vi "Loop_SM.vi"() -> ()   [LabVIEW 2017, in "Claw_Rotation.lvlib"]
uses:
  Claw_Rotation.lvlib
  CLUSTER_CMD_SM_Lift_Rotate.ctl
  ENUM_SM_Rotate_Positions.ctl
  _SHARE ALL/TypeDef Share All/CLUSTER_TalonInput.ctl
  System Drivers/Phoenix-LabVIEW/Motor Controller/Controls/CTRE_Phoenix_MotorControl_ControlMode.ctl
  TypeDef/CLUSTER_PID.ctl
  ENUM_SM_State.ctl
  CLUSTER_ACT_Lift Output.ctl
  _SHARE ALL/RoboRio Share All/SRX Share All/TypeDefs SRX/Cluster_SRX_General Data.ctl
  _SHARE ALL/RoboRio Share All/SRX Share All/TypeDefs SRX/Cluster_SRX_Common Runtime Data.ctl
  _SHARE ALL/RoboRio Share All/SRX Share All/TypeDefs SRX/Cluster_SRX_Error Calculations.ctl
  _SHARE ALL/RoboRio Share All/SRX Share All/TypeDefs SRX/Cluster_SRX_Voltage Out Data.ctl
  _SHARE ALL/RoboRio Share All/SRX Share All/TypeDefs SRX/Cluster_SRX_Sensor Out Data.ctl
  _SHARE ALL/RoboRio Share All/SRX Share All/TypeDefs SRX/Cluster_SRX_Sensor Quad Data.ctl
  _SHARE ALL/RoboRio Share All/SRX Share All/TypeDefs SRX/Cluster_SRX_Analog In Data.ctl
  _SHARE ALL/RoboRio Share All/SRX Share All/TypeDefs SRX/Cluster_SRX_PWM Sensor Data.ctl
  _SHARE ALL/RoboRio Share All/SRX Share All/TypeDefs SRX/Cluster_SRX_F and R Limit Indicators.ctl
  ENUM_SM_Action.ctl
  Globals/Global_Device_IDs.vi
  _SHARE ALL/Global Share All/Global_STOP.vi
  Global_CMD.vi
  Global_ACT Write_Data Out.vi
  Global_SM Write_Data Out.vi
panel:
  out "State":T1
  out "SM Output":T2 {"Talon Mode" items=["PercentOutput"=0, "Position"=1, "Velocity"=2, "Current"=3, "Follower"=5, "MotionProfile"=6, "MotionMagic"=7, "MotionMagicArc"=8, "MotionProfileArc"=10, "Disabled"=15]}
  out "SM CMD Input":T5={"Enable System"=TRUE, "Rotate Position"=enum."Starting: 0", "Manual Velocity"=0.0, "Manual Mode"=FALSE}
  out "Cycle Time (S)":dbl format="%.3g"
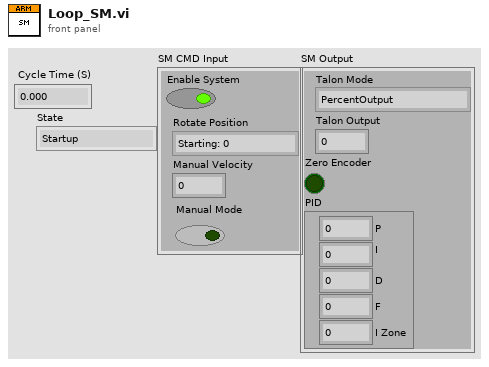
[diagram p1: front panel]
types:
  T1 = typedef "Claw_Rotation.lvlib/ENUM_SM_State.ctl" = enum16{"Startup", "Idle", "Manual", "Position - Moving", "Position - Holding", "Shutdown"}
  T2 = typedef "CLUSTER_TalonInput.ctl" = cluster{"Talon Mode":T3, "Talon Output":dbl, "Zero Encoder":bool, "PID":T4}
  T3 = typedef "CTRE_Phoenix_MotorControl_ControlMode.ctl" = u16
  T4 = typedef "CLUSTER_PID.ctl" = cluster{"P":dbl, "I":dbl, "D":dbl, "F":dbl, "I Zone":dbl}
  T5 = typedef "Claw_Rotation.lvlib/CLUSTER_CMD_SM_Lift_Rotate.ctl" = cluster{"Enable System":bool, "Rotate Position":T6, "Manual Velocity":dbl, "Manual Mode":bool}
  T6 = typedef "Claw_Rotation.lvlib/ENUM_SM_Rotate_Positions.ctl" = enum16{"Starting: 0"}
  T7 = typedef "Claw_Rotation.lvlib/CLUSTER_ACT_Lift Output.ctl" = cluster{"Device Info Out":T8, "Common Runtime Data Out":T9, "Quad Sensor Data Out":T13, "Analog Sensor Data Out":T14, "PWM Data Out":T15, "Hard Limits Out":T16}
  T8 = typedef "Cluster_SRX_General Data.ctl" = cluster{"Device ID":i32, "Firmware Version":i32, "Inverted?":bool, "Has Reset Occurred?":bool}
  T9 = typedef "Cluster_SRX_Common Runtime Data.ctl" = cluster{"Calc":T10, "Voltage ":T11, "Sensor":T12, "Current":dbl, "Temp":dbl}
  T10 = typedef "Cluster_SRX_Error Calculations.ctl" = cluster{"Error":i32, "D-Error":dbl, "I-Acc":dbl}
  T11 = typedef "Cluster_SRX_Voltage Out Data.ctl" = cluster{"Percent":dbl, "Output":dbl, "Bus":dbl}
  T12 = typedef "Cluster_SRX_Sensor Out Data.ctl" = cluster{"Pos":i32, "Vel":i32}
  T13 = typedef "Cluster_SRX_Sensor Quad Data.ctl" = cluster{"Position":i32, "Velocity":i32, "Quad A Pin":bool, "Quad B Pin":bool, "Quad Idx Pin":bool}
  T14 = typedef "Cluster_SRX_Analog In Data.ctl" = cluster{"WithOv":i32, "Raw":i32, "Velocity":i32}
  T15 = typedef "Cluster_SRX_PWM Sensor Data.ctl" = cluster{"Position":i32, "Velocity":i32, "High(us)":i32, "Period(us)":i32}
  T16 = typedef "Cluster_SRX_F and R Limit Indicators.ctl" = cluster{"Forward Closed?":bool, "Reverse Closed?":bool}
  T17 = typedef "Claw_Rotation.lvlib/ENUM_SM_Action.ctl" = enum16{"No Action", "Reset Time", "Reset All", "Reset Encoder", "Manual", "Position", "Set PID 1", "Disable Motor"}
  T18 = typedef "CLUSTER_Arm_Device_IDs.ctl" = cluster{"Master":T19, "Slave":T19}
  T19 = typedef "CLUSTER_Talon_Setup.ctl" = cluster{"Open Data":T20, "Current Config Data":T21, "Sensor Config":T22, "Hard Limits":T24, "Motion Magic Config Data":T26, "PIDF":T27, "Maximum Integral Accumulator Value":dbl, "AllowableClosedLoop":i32, "Limits":T28, "Output Config":T29}
  T20 = typedef "Cluster_SRX_OPEN Data.ctl" = cluster{"SRX ID":u8, "Invert Output":bool}
  T21 = typedef "Cluster_SRX_Current Config.ctl" = cluster{"Enable Current Limit?":bool, "Peak Current (Amps)":i32, "Peak Current Maximum Duration (ms)":i32, "Continuous Current Limit (Amps)":i32}
  T22 = typedef "Cluster_SRX_Sensor Config.ctl" = cluster{"Feedback Device":T23, "PhaseSensor":bool}
  T23 = typedef "CTRE_Phoenix_MotorControl_FeedbackDevice.ctl" = i8
  T24 = typedef "Cluster_SRX_Config Hard Limits.ctl" = cluster{"Fwd Enable":bool, "Rev Enable":bool, "Fwd NO-NC":T25, "Rev NO-NC":T25}
  T25 = typedef "CTRE_Phoenix_MotorControl_LimitSwitchNormal.ctl" = enum16{"Normally Open", "Normally Closed", "Disabled"}
  T26 = typedef "Cluster_SRX_Motion Magic Config Data.ctl" = cluster{"Cruise Velocity":i32, "Acceleration":i32}
  T27 = typedef "Cluster_SRX_PIDF.ctl" = cluster{"P":dbl, "I":dbl, "D":dbl, "F":dbl, "I Zone":dbl}
  T28 = typedef "Cluster_SRX_Config Soft Limits.ctl" = cluster{"Max":i32, "Min":i32, "Max Enable":bool, "Min Enable":bool}
  T29 = typedef "Cluster_SRX_Config Voltage Output.ctl" = cluster{"Invert?":bool, "Neutral Mode":T30, "Deadband (-1to1)":dbl, "Ramp Time Off to Full (S)":dbl, "Peak  (-1to1)":T31, "Nominal  (-1to1)":T31}
  T30 = typedef "CTRE_Phoenix_MotorControl_NeutralMode.ctl" = enum8{"EEPROMSetting", "Override to Coast", "Override to Brake"}
  T31 = typedef "Cluster_SRX_Forward and Reverse.ctl" = cluster{"Forward":dbl, "Reverse":dbl}
  T32 = cluster{"State":T1, "Previous State":T1, "Current Time":timestamp, "Previous Time":timestamp, "Start Time":timestamp, "Target Time (ms)":u32, "Cycle Time(S)":dbl, "Arm_Output":T7, "SM CMD Input":T5, "SM Output":T2, "Lift Setup":T18}
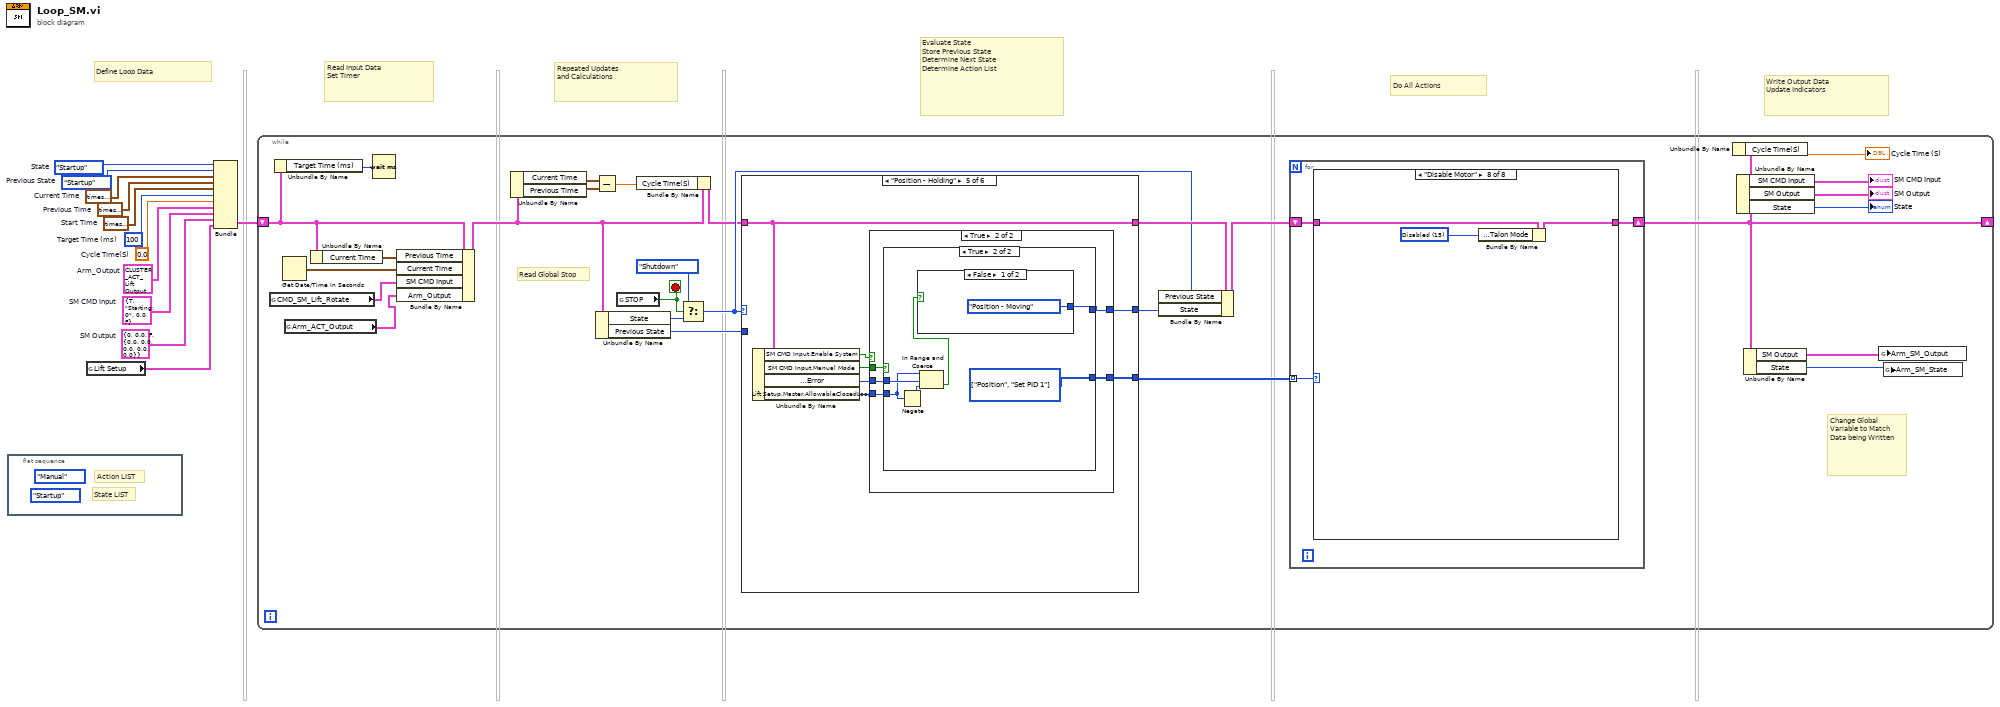
[diagram p0: block diagram]
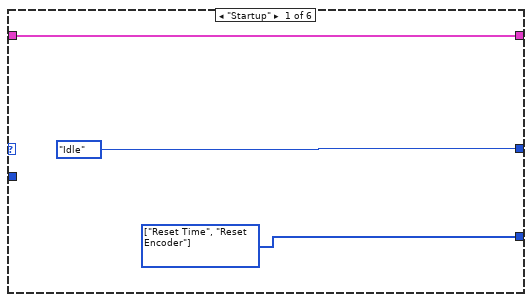
[diagram p2: hidden frame]
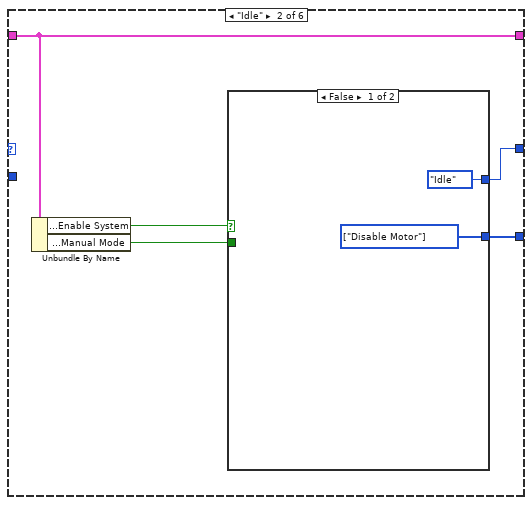
[diagram p3: hidden frame]
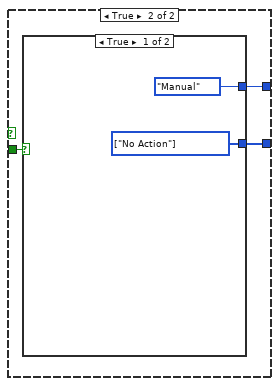
[diagram p4: hidden frame]
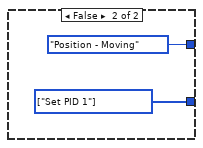
[diagram p5: hidden frame]
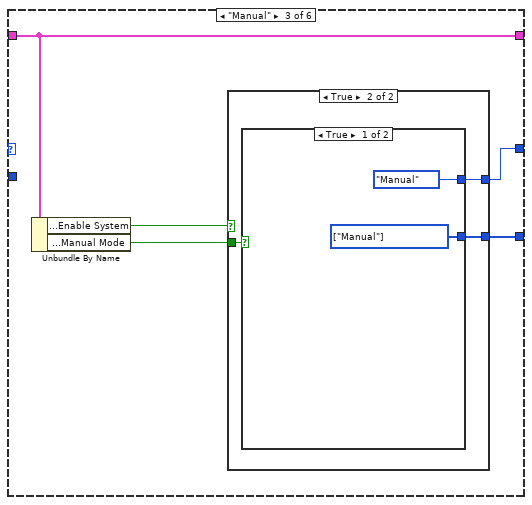
[diagram p6: hidden frame]
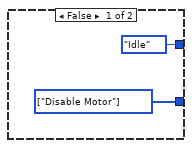
[diagram p7: hidden frame]
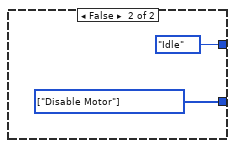
[diagram p8: hidden frame]
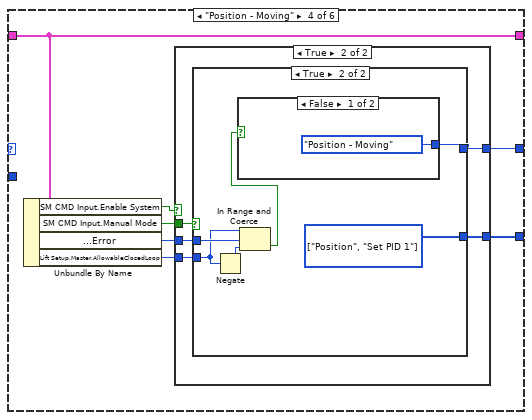
[diagram p9: hidden frame]
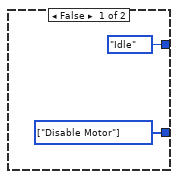
[diagram p10: hidden frame]
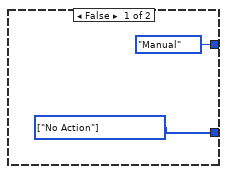
[diagram p11: hidden frame]
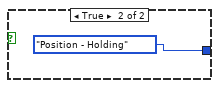
[diagram p12: hidden frame]
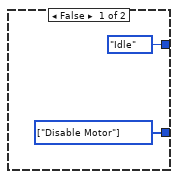
[diagram p13: hidden frame]
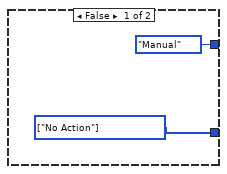
[diagram p14: hidden frame]
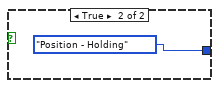
[diagram p15: hidden frame]
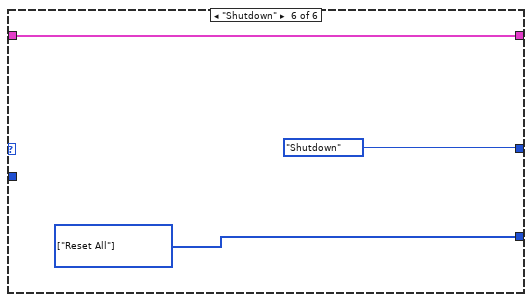
[diagram p16: hidden frame]
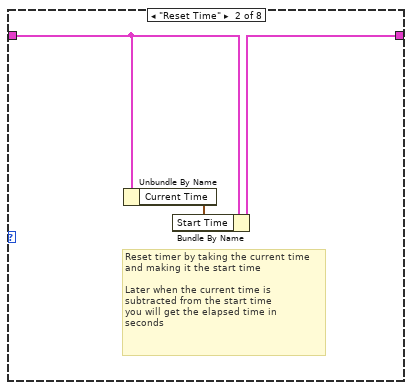
[diagram p18: hidden frame]
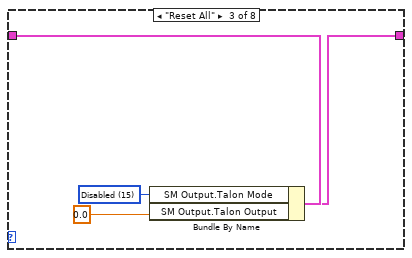
[diagram p19: hidden frame]
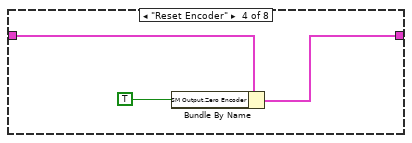
[diagram p20: hidden frame]
diagram:
  w2 = T2 {"Talon Mode"=0, "Talon Output"=0.0, "Zero Encoder"=FALSE, "PID"={"P"=0.0, "I"=0.0, "D"=0.0, "F"=0.0, "I Zone"=0.0}}  # SM Output
  w3 = T5 {"Enable System"=TRUE, "Rotate Position"=enum."Starting: 0", "Manual Velocity"=0.0, "Manual Mode"=FALSE}  # SM CMD Input
  w4 = T7 {"Device Info Out"={"Device ID"=0, "Firmware Version"=0, "Inverted?"=FALSE, "Has Reset Occurred?"=FALSE}, "Common Runtime Data Out"={"Calc"={"Error"=0, "D-Error"=0.0, "I-Acc"=0.0}, "Voltage "={"Percent"=0.0, "Output"=0.0, "Bus"=0.0}, "Sensor"={"Pos"=0, "Vel"=0}, "Current"=0.0, "Temp"=0.0}, "Quad Sensor Data Out"={"Position"=0, "Velocity"=0, "Quad A Pin"=FALSE, "Quad B Pin"=FALSE, "Quad Idx Pin"=FALSE}, "Analog Sensor Data Out"={"WithOv"=0, "Raw"=0, "Velocity"=0}, "PWM Data Out"={"Position"=0, "Velocity"=0, "High(us)"=0, "Period(us)"=0}, "Hard Limits Out"={"Forward Closed?"=FALSE, "Reverse Closed?"=FALSE}}  # Arm_Output
  w5 = 0.0  # Cycle Time(S)
  w6 = ENUM_SM_State."Startup"  # Previous State
  w7 = timestamp(0 s since 1904-01-01)  # Previous Time
  w8 = u32 100  # Target Time (ms)
  w9 = timestamp(0 s since 1904-01-01)  # Start Time
  w10 = timestamp(0 s since 1904-01-01)  # Current Time
  w11 = ENUM_SM_State."Startup"  # State
  # "Define Loop Data"
  # "Repeated Updates\nand Calculations"
  # "Read Input Data\nSet Timer"
  # "Evaluate State\nStore Previous State\nDetermine Next State\nDetermine Action List"
  # "Do All Actions"
  # "Write Output Data\nUpdate Indicators"
  n1 = flat-sequence {
    frame #0 {
      (unwired) ENUM_SM_State."Startup" ("State")
      (unwired) ENUM_SM_Action."Manual" ("Action")
      # "State LIST"
      # "Action LIST"
    }
  }
  n2 = global read "Global_Device_IDs.vi" "Lift Setup"() -> (w1:T18)
  n3 = Bundle("State"=w11, "Previous State"=w6, "Current Time"=w10, "Previous Time"=w7, "Start Time"=w9, "Target Time (ms)"=w8, "Cycle Time(S)"=w5, "Arm_Output"=w4, "SM CMD Input"=w3, "SM Output"=w2, "Lift Setup"=w1) -> (w12:T32)  [unwired: 1 in]
  n4 = while {
    shift-right: [w28] -> _
    shift-left: w12 -> [w31]
    stop <- w36 stop-if-true
    # "Change Global\nVariable to Match\nData being Written"
    # "Read Global Stop"
    n5 = global read "Global_CMD.vi" "CMD_SM_Lift_Rotate"() -> (w20:T5)
    n6 = Unbundle By Name(w31) -> ("Target Time (ms)"=w33:u32)
    n7 = Get Date/Time In Seconds() -> (seconds since 1Jan1904=w39:timestamp)
    n8 = global read "Global_ACT Write_Data Out.vi" "Arm_ACT_Output"() -> (w19:T7)
    n9 = Unbundle By Name(w31) -> ("Current Time"=w32:timestamp)
    n10 = Wait (ms)(milliseconds to wait=w33) -> ()  [unwired: 1 out]
    n11 = Bundle By Name(cluster=w31, "Previous Time"=w32, "Current Time"=w39, "SM CMD Input"=w20, "Arm_Output"=w19) -> (w24:T32)
    n12 = Unbundle By Name(w24) -> ("Current Time"=w25:timestamp, "Previous Time"=w26:timestamp)
    n13 = Subtract(x=w25, y=w26) -> (x-y=w22:dbl)
    n14 = Unbundle By Name(w24) -> ("State"=w34:T1, "Previous State"=w30:T1)
    n15 = global read "Global_STOP.vi" "STOP"() -> (w36:bool)
    n16 = Bundle By Name(cluster=w24, "Cycle Time(S)"=w22) -> (w23:T32)
    n17 = Select(t=ENUM_SM_State."Shutdown" ("State"), s=w36, f=w34) -> (s? t:f=w29:T1)
    n18 = case shown="\"Position - Holding\"" w29 {
      tunnel: w23 -> [w42 w47 w61 w77 w101 w121]
      tunnel: [w42 w47 w61 w77 w101 w121] -> w37
      tunnel: [w41 w43 w57 w73 w97 w120] -> w21
      tunnel: w30 -> [_ _ _ _ _ _]
      tunnel: [ENUM_SM_State."Idle" ("State") w44 w58 w72 w96 ENUM_SM_State."Shutdown" ("State")] -> w18
      frame "Startup" {
        w41 = T17[] [enum."Reset Time", enum."Reset Encoder"] items=["No Action", "Reset Time", "Reset All", "Reset Encoder", "Manual", "Position", "Set PID 1", "Disable Motor"] ("Actions")
      }
      frame "Idle" {
        n19 = Unbundle By Name(w47) -> ("SM CMD Input.Enable System"=w46:bool, "SM CMD Input.Manual Mode"=w45:bool)
        n20 = case shown="False" w46 {
          tunnel: w45 -> [_ w52]
          tunnel: [ENUM_SM_State."Idle" ("State") w51] -> w44
          tunnel: [w48 w50] -> w43
          frame False {
            w48 = T17[] [enum."Disable Motor"] items=["No Action", "Reset Time", "Reset All", "Reset Encoder", "Manual", "Position", "Set PID 1", "Disable Motor"] ("Actions")
          }
          frame True {
            n21 = case shown="True" w52 {
              tunnel: [ENUM_SM_State."Manual" ("State") ENUM_SM_State."Position - Moving" ("State")] -> w51
              tunnel: [w53 w55] -> w50
              frame True {
                w53 = T17[] [enum."No Action"] items=["No Action", "Reset Time", "Reset All", "Reset Encoder", "Manual", "Position", "Set PID 1", "Disable Motor"] ("Actions")
              }
              frame False {
                w55 = T17[] [enum."Set PID 1"] items=["No Action", "Reset Time", "Reset All", "Reset Encoder", "Manual", "Position", "Set PID 1", "Disable Motor"] ("Actions")
              }
            }
          }
        }
      }
      frame "Manual" {
        n22 = Unbundle By Name(w61) -> ("SM CMD Input.Enable System"=w60:bool, "SM CMD Input.Manual Mode"=w59:bool)
        n23 = case shown="True" w60 {
          tunnel: w59 -> [_ w66]
          tunnel: [ENUM_SM_State."Idle" ("State") w65] -> w58
          tunnel: [w62 w64] -> w57
          frame False {
            w62 = T17[] [enum."Disable Motor"] items=["No Action", "Reset Time", "Reset All", "Reset Encoder", "Manual", "Position", "Set PID 1", "Disable Motor"] ("Actions")
          }
          frame True {
            n24 = case shown="True" w66 {
              tunnel: [ENUM_SM_State."Manual" ("State") ENUM_SM_State."Idle" ("State")] -> w65
              tunnel: [w67 w69] -> w64
              frame True {
                w67 = T17[] [enum."Manual"] items=["No Action", "Reset Time", "Reset All", "Reset Encoder", "Manual", "Position", "Set PID 1", "Disable Motor"] ("Actions")
              }
              frame False {
                w69 = T17[] [enum."Disable Motor"] items=["No Action", "Reset Time", "Reset All", "Reset Encoder", "Manual", "Position", "Set PID 1", "Disable Motor"] ("Actions")
              }
            }
          }
        }
      }
      frame "Position - Moving" {
        n25 = Unbundle By Name(w77) -> ("SM CMD Input.Enable System"=w71:bool, "SM CMD Input.Manual Mode"=w76:bool, "Arm_Output.Common Runtime Data Out.Calc.Error"=w75:i32, "Lift Setup.Master.AllowableClosedLoop"=w74:i32)
        n26 = case shown="True" w71 {
          tunnel: w76 -> [_ w84]
          tunnel: w75 -> [_ w83]
          tunnel: w74 -> [_ w82]
          tunnel: [w78 w81] -> w73
          tunnel: [ENUM_SM_State."Idle" ("State") w80] -> w72
          frame False {
            w78 = T17[] [enum."Disable Motor"] items=["No Action", "Reset Time", "Reset All", "Reset Encoder", "Manual", "Position", "Set PID 1", "Disable Motor"] ("Actions")
          }
          frame True {
            n27 = case shown="True" w84 {
              tunnel: w83 -> [_ w92]
              tunnel: w82 -> [_ w91]
              tunnel: [w85 w88] -> w81
              tunnel: [ENUM_SM_State."Manual" ("State") w87] -> w80
              frame False {
                w85 = T17[] [enum."No Action"] items=["No Action", "Reset Time", "Reset All", "Reset Encoder", "Manual", "Position", "Set PID 1", "Disable Motor"] ("Actions")
              }
              frame True {
                w88 = T17[] [enum."Position", enum."Set PID 1"] items=["No Action", "Reset Time", "Reset All", "Reset Encoder", "Manual", "Position", "Set PID 1", "Disable Motor"] ("Actions")
                n28 = Negate(x=w91) -> (-x=w90:i32)
                n29 = In Range and Coerce(upper limit=w91, x=w92, lower limit=w90) -> (In Range?=w89:bool)  [unwired: 1 out]
                n30 = case shown="False" w89 {
                  tunnel: [ENUM_SM_State."Position - Moving" ("State") ENUM_SM_State."Position - Holding" ("State")] -> w87
                  frame False {
                  }
                  frame True {
                  }
                }
              }
            }
          }
        }
      }
      frame "Position - Holding" {
        n31 = Unbundle By Name(w101) -> ("SM CMD Input.Enable System"=w95:bool, "SM CMD Input.Manual Mode"=w100:bool, "Arm_Output.Common Runtime Data Out.Calc.Error"=w99:i32, "Lift Setup.Master.AllowableClosedLoop"=w98:i32)
        n32 = case shown="True" w95 {
          tunnel: w100 -> [_ w108]
          tunnel: w99 -> [_ w107]
          tunnel: w98 -> [_ w106]
          tunnel: [w102 w105] -> w97
          tunnel: [ENUM_SM_State."Idle" ("State") w104] -> w96
          frame False {
            w102 = T17[] [enum."Disable Motor"] items=["No Action", "Reset Time", "Reset All", "Reset Encoder", "Manual", "Position", "Set PID 1", "Disable Motor"] ("Actions")
          }
          frame True {
            n33 = case shown="True" w108 {
              tunnel: w107 -> [_ w116]
              tunnel: w106 -> [_ w115]
              tunnel: [w109 w112] -> w105
              tunnel: [ENUM_SM_State."Manual" ("State") w111] -> w104
              frame False {
                w109 = T17[] [enum."No Action"] items=["No Action", "Reset Time", "Reset All", "Reset Encoder", "Manual", "Position", "Set PID 1", "Disable Motor"] ("Actions")
              }
              frame True {
                w112 = T17[] [enum."Position", enum."Set PID 1"] items=["No Action", "Reset Time", "Reset All", "Reset Encoder", "Manual", "Position", "Set PID 1", "Disable Motor"] ("Actions")
                n34 = Negate(x=w115) -> (-x=w114:i32)
                n35 = In Range and Coerce(upper limit=w115, x=w116, lower limit=w114) -> (In Range?=w113:bool)  [unwired: 1 out]
                n36 = case shown="False" w113 {
                  tunnel: [ENUM_SM_State."Position - Moving" ("State") ENUM_SM_State."Position - Holding" ("State")] -> w111
                  frame False {
                  }
                  frame True {
                  }
                }
              }
            }
          }
        }
      }
      frame "Shutdown" {
        w120 = T17[] [enum."Reset All"] items=["No Action", "Reset Time", "Reset All", "Reset Encoder", "Manual", "Position", "Set PID 1", "Disable Motor"] ("Actions")
      }
    }
    n37 = Bundle By Name(cluster=w37, "Previous State"=w29, "State"=w18) -> (w38:T32)
    n38 = for {
      tunnel: w21 -> [w124] mode=indexing
      shift-right: [w123] -> w28
      shift-left: w38 -> [w122]
      n39 = case shown="\"Disable Motor\"" w124 {
        tunnel: w122 -> [w125 w128 w132 w135 w140 w155 w158 w162]
        tunnel: [w125 w127 w131 w134 w139 w156 w159 w161] -> w123
        frame "No Action" {
        }
        frame "Reset Time" {
          # "Reset timer by taking the current time\nand making it the start time\n\nLater when the current time is \nsubtracted from the start time\nyou will get the elapsed time in \nseconds"
          n40 = Unbundle By Name(w128) -> ("Current Time"=w126:timestamp)
          n41 = Bundle By Name(cluster=w128, "Start Time"=w126) -> (w127:T32)
        }
        frame "Reset All" {
          w130 = T3 15 items=["PercentOutput"=0, "Position"=1, "Velocity"=2, "Current"=3, "Follower"=5, "MotionProfile"=6, "MotionMagic"=7, "MotionMagicArc"=8, "MotionProfileArc"=10, "Disabled"=15] ("SM Output.Talon Mode")
          n42 = Bundle By Name(cluster=w132, "SM Output.Talon Mode"=w130, "SM Output.Talon Output"=0.0) -> (w131:T32)
        }
        frame "Reset Encoder" {
          n43 = Bundle By Name(cluster=w135, "SM Output.Zero Encoder"=TRUE) -> (w134:T32)
        }
        frame "Manual" {
          n44 = Unbundle By Name(w140) -> ("SM CMD Input.Manual Velocity"=w138:dbl, "Lift Setup.Master.Output Config.Deadband (-1to1)"=w143:dbl)
          n45 = Negate(x=w143) -> (-x=w142:dbl)
          n46 = In Range and Coerce(upper limit=w143, x=w138, lower limit=w142) -> (In Range?=w141:bool)  [unwired: 1 out]
          n47 = case shown="False" w141 {
            tunnel: w138 -> [_ w146]
            tunnel: [w145 w147] -> w137
            tunnel: [0.0 w146] -> w136
            frame True {
              w145 = T3 15 items=["PercentOutput"=0, "Position"=1, "Velocity"=2, "Current"=3, "Follower"=5, "MotionProfile"=6, "MotionMagic"=7, "MotionMagicArc"=8, "MotionProfileArc"=10, "Disabled"=15] ("SM Output.Talon Mode")
            }
            frame False {
              w147 = T3 0 items=["PercentOutput"=0, "Position"=1, "Velocity"=2, "Current"=3, "Follower"=5, "MotionProfile"=6, "MotionMagic"=7, "MotionMagicArc"=8, "MotionProfileArc"=10, "Disabled"=15] ("SM Output.Talon Mode")
            }
          }
          n48 = Bundle By Name(cluster=w140, "SM Output.Talon Mode"=w137, "SM Output.Talon Output"=w136) -> (w139:T32)
        }
        frame "Position" {
          n49 = Unbundle By Name(w155) -> ("SM CMD Input.Rotate Position"=w149:T6)
          n50 = Format Into String(w149) -> (resulting string=w154:string)  [unwired: 3 in, 1 out]
          n51 = Match Pattern(string=w154, regular expression=":") -> (before substring=w152:string, after substring=w151:string)  [unwired: 1 in, 2 out]
          n52 = call <vilib>:"Trim Whitespace.vi"("string"=w152) -> ()  [unwired: 1 in, 1 out]
          n53 = call <vilib>:"Trim Whitespace.vi"("string"=w151) -> ("trimmed string"=w150:string)  [unwired: 1 in]
          n54 = Decimal String To Number(string=w150) -> (number=w148:i32)  [unwired: 2 in, 1 out]
          n55 = Bundle By Name(cluster=w155, "SM Output.Talon Output"=w148) -> (w156:T32)
        }
        frame "Set PID 1" {
          n56 = Unbundle By Name(w158) -> ("Lift Setup.Master.PIDF"=w157:T27)
          n57 = Bundle By Name(cluster=w158, "SM Output.PID"=w157) -> (w159:T32)
        }
        frame "Disable Motor" {
          w160 = T3 15 items=["PercentOutput"=0, "Position"=1, "Velocity"=2, "Current"=3, "Follower"=5, "MotionProfile"=6, "MotionMagic"=7, "MotionMagicArc"=8, "MotionProfileArc"=10, "Disabled"=15] ("SM Output.Talon Mode")
          n58 = Bundle By Name(cluster=w162, "SM Output.Talon Mode"=w160) -> (w161:T32)
        }
      }
    }
    n59 = Unbundle By Name(w28) -> ("Cycle Time(S)"=→"Cycle Time (S)":dbl)
    n60 = Unbundle By Name(w28) -> ("SM CMD Input"=→"SM CMD Input":T5, "SM Output"=→"SM Output":T2, "State"=→"State":T1)
    n61 = Unbundle By Name(w28) -> ("SM Output"=w16:T2, "State"=w17:T1)
    n62 = global write "Global_SM Write_Data Out.vi" "Arm_SM_Output"(w16) -> ()
    n63 = global write "Global_SM Write_Data Out.vi" "Arm_SM_State"(w17) -> ()
  }
